vi "Popup - Select Operation.vi"(8 "error in (no error)":errorcluster, 11 "Controller (Host) Data in":T2={"State"=enum."APU Select", "2D User Info"=[], "APU Setup File"={"Sensor Info"=[], "Variables"=[], "CMM Table 106"=[], "CMM Table 106B "=[], "Accel Config"=[], "Report Sheet 1"=[], "Report Sheet 2"=[], "Report Sheet 3"=[]}, "Test Information"={"APU Part Number:"="", "Model:"="", "Serial Number:"="", "Customer:"="", "Work Order:"="", "Pre or Post SB"="", "Run Count"=0, "APU Selected"="<Select>"}, "ChannelTags"=[], "Live_Min_Max_Dev"=[], "CalChannels"=[], "Slopes"=[], "Offsets"=[], "Calculated Values"={"C.00"=0.0, "C.01"=0.0, "C.02"=0.0, "C.03"=0.0, "C.04"=0.0, "C.05"=0.0, "C.06"=0.0, "C.07"=0.0, "C.08"=0.0, "C.09"=0.0, "C.10"=0.0, "C.11"=0.0, "C.12"=0.0, "C.13"=0.0, "C.14"=0.0, "C.15"=0.0, "C.16"=0.0, "C.17"=0.0, "C.18"=0.0, "C.19"=0.0, "C.20"=0.0, "C.21"=0.0, "C.22"=0.0, "C.23"=0.0, "C.24"=0.0, "C.25"=0.0, "C.26"=0.0, "C.27"=0.0, "C.28"=0.0, "C.29"=0.0, "C.30"=0.0, "C.31"=0.0, "C.32"=0.0, "C.33"=0.0, "C.34"=0.0, "C.35"=0.0, "C.36"=0.0, "C.37"=0.0, "C.38"=0.0, "C.39"=0.0, "C.40"=0.0, "C.41"=0.0, "C.42"=0.0, "C.43"=0.0, "C.44"=0.0, "C.45"=0.0, "C.46"=0.0, "C.47"=0.0, "C.48"=0.0, "C.49"=0.0, "C.50"=0.0, "C.51"=0.0, "C.52"=0.0, "C.53"=0.0, "C.54"=0.0, "C.55"=0.0, "C.56"=0.0, "C.57"=0.0, "C.58"=0.0, "C.59"=0.0, "C.60"=0.0, "C.61"=0.0, "C.62"=0.0}, "ThresholdChannels"=[], "ThresholdRPM"=[], "ThresholdMin"=[], "ThresholdValue"=[], "HeavyCCM"=[], "LightCCM"=[], "FuelFarm"=FALSE} {"Test Information"."Run Count" min=0 step=1}) -> (0 "error out":errorcluster, 3 "Controller (Host) Data out":T2={"State"=enum."APU Select", "2D User Info"=[], "APU Setup File"={"Sensor Info"=[], "Variables"=[], "CMM Table 106"=[], "CMM Table 106B "=[], "Accel Config"=[], "Report Sheet 1"=[], "Report Sheet 2"=[], "Report Sheet 3"=[]}, "Test Information"={"APU Part Number:"="", "Model:"="", "Serial Number:"="", "Customer:"="", "Work Order:"="", "Pre or Post SB"="", "Run Count"=0, "APU Selected"="<Select>"}, "ChannelTags"=[], "Live_Min_Max_Dev"=[], "CalChannels"=[], "Slopes"=[], "Offsets"=[], "Calculated Values"={"C.00"=0.0, "C.01"=0.0, "C.02"=0.0, "C.03"=0.0, "C.04"=0.0, "C.05"=0.0, "C.06"=0.0, "C.07"=0.0, "C.08"=0.0, "C.09"=0.0, "C.10"=0.0, "C.11"=0.0, "C.12"=0.0, "C.13"=0.0, "C.14"=0.0, "C.15"=0.0, "C.16"=0.0, "C.17"=0.0, "C.18"=0.0, "C.19"=0.0, "C.20"=0.0, "C.21"=0.0, "C.22"=0.0, "C.23"=0.0, "C.24"=0.0, "C.25"=0.0, "C.26"=0.0, "C.27"=0.0, "C.28"=0.0, "C.29"=0.0, "C.30"=0.0, "C.31"=0.0, "C.32"=0.0, "C.33"=0.0, "C.34"=0.0, "C.35"=0.0, "C.36"=0.0, "C.37"=0.0, "C.38"=0.0, "C.39"=0.0, "C.40"=0.0, "C.41"=0.0, "C.42"=0.0, "C.43"=0.0, "C.44"=0.0, "C.45"=0.0, "C.46"=0.0, "C.47"=0.0, "C.48"=0.0, "C.49"=0.0, "C.50"=0.0, "C.51"=0.0, "C.52"=0.0, "C.53"=0.0, "C.54"=0.0, "C.55"=0.0, "C.56"=0.0, "C.57"=0.0, "C.58"=0.0, "C.59"=0.0, "C.60"=0.0, "C.61"=0.0, "C.62"=0.0}, "ThresholdChannels"=[], "ThresholdRPM"=[], "ThresholdMin"=[], "ThresholdValue"=[], "HeavyCCM"=[], "LightCCM"=[], "FuelFarm"=FALSE} {"Test Information"."Run Count" min=0 step=1})   [LabVIEW 2018, in "Controller (Host).lvlib"]
doc: "This is the dialog used by the user to select an operation to perform."
uses:
  Controller (Host).lvlib
  Private Controls/Controller (Host) Data.ctl
  Private Controls/State.ctl
  Top Level/Shared Controls/APU Setup File.ctl
  Public Controls/Test Information.ctl
  Public VIs/PreorPostSB.ctl
  Public Controls/APU Select.ctl
  Top Level/Shared Controls/Calculated Data.ctl
  File IO/Public Controls/Variables.ctl
  File IO/File IO.lvlib
  Testing UI 1/Testing UI 1.lvlib
panel:
  in  "Revert":bool
  in  "Variables":T1
  out "APU Selected":string
  in  "Confirm":bool
  # "Change APU Variables:"
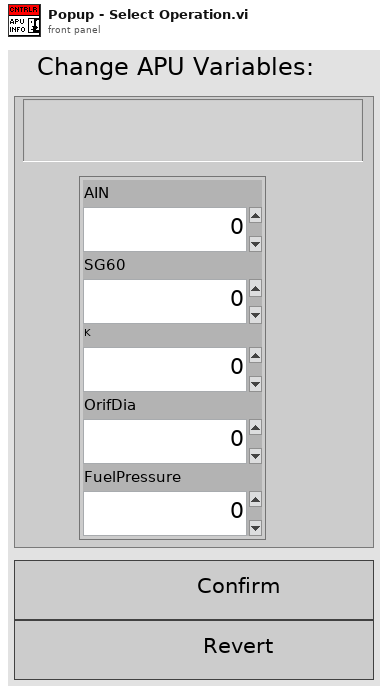
[diagram p1: front panel]
types:
  T1 = typedef "File IO.lvlib/Variables.ctl" = cluster{"AIN":dbl, "SG60":dbl, "K":dbl, "OrifDia":dbl, "FuelPressure":dbl}
  T2 = typedef "Controller (Host).lvlib/Controller (Host) Data.ctl" = cluster{"State":T3, "2D User Info":string[][], "APU Setup File":T4, "Test Information":T5, "ChannelTags":string[], "Live_Min_Max_Dev":dbl[][], "CalChannels":string[], "Slopes":dbl[], "Offsets":dbl[], "Calculated Values":T8, "ThresholdChannels":string[], "ThresholdRPM":dbl[], "ThresholdMin":bool[], "ThresholdValue":dbl[], "HeavyCCM":dbl[][], "LightCCM":dbl[][], "FuelFarm":bool}
  T3 = typedef "Controller (Host).lvlib/State.ctl" = enum16{"APU Select", "Operation Select", "SubTests Select", "Calibration", "Testing", "Exit"}
  T4 = typedef "APU Setup File.ctl" = cluster{"Sensor Info":string[][], "Variables":string[][], "CMM Table 106":string[][], "CMM Table 106B ":string[][], "Accel Config":string[][], "Report Sheet 1":string[][], "Report Sheet 2":string[][], "Report Sheet 3":string[][]}
  T5 = typedef "Controller (Host).lvlib/Test Information.ctl" = cluster{"APU Part Number:":string, "Model:":string, "Serial Number:":string, "Customer:":string, "Work Order:":string, "Pre or Post SB":T6, "Run Count":i32, "APU Selected":T7}
  T6 = typedef "Controller (Host).lvlib/PreorPostSB.ctl" = string
  T7 = typedef "Controller (Host).lvlib/APU Select.ctl" = string
  T8 = typedef "Calculated Data.ctl" = cluster{"C.00":dbl, "C.01":dbl, "C.02":dbl, "C.03":dbl, "C.04":dbl, "C.05":dbl, "C.06":dbl, "C.07":dbl, "C.08":dbl, "C.09":dbl, "C.10":dbl, "C.11":dbl, "C.12":dbl, "C.13":dbl, "C.14":dbl, "C.15":dbl, "C.16":dbl, "C.17":dbl, "C.18":dbl, "C.19":dbl, "C.20":dbl, "C.21":dbl, "C.22":dbl, "C.23":dbl, "C.24":dbl, "C.25":dbl, "C.26":dbl, "C.27":dbl, "C.28":dbl, "C.29":dbl, "C.30":dbl, "C.31":dbl, "C.32":dbl, "C.33":dbl, "C.34":dbl, "C.35":dbl, "C.36":dbl, "C.37":dbl, "C.38":dbl, "C.39":dbl, "C.40":dbl, "C.41":dbl, "C.42":dbl, "C.43":dbl, "C.44":dbl, "C.45":dbl, "C.46":dbl, "C.47":dbl, "C.48":dbl, "C.49":dbl, "C.50":dbl, "C.51":dbl, "C.52":dbl, "C.53":dbl, "C.54":dbl, "C.55":dbl, "C.56":dbl, "C.57":dbl, "C.58":dbl, "C.59":dbl, "C.60":dbl, "C.61":dbl, "C.62":dbl}
  T9 = cluster{"AIN":bool, "SG60":bool, "K":bool, "OrifDia":bool, "FuelPressure":bool}
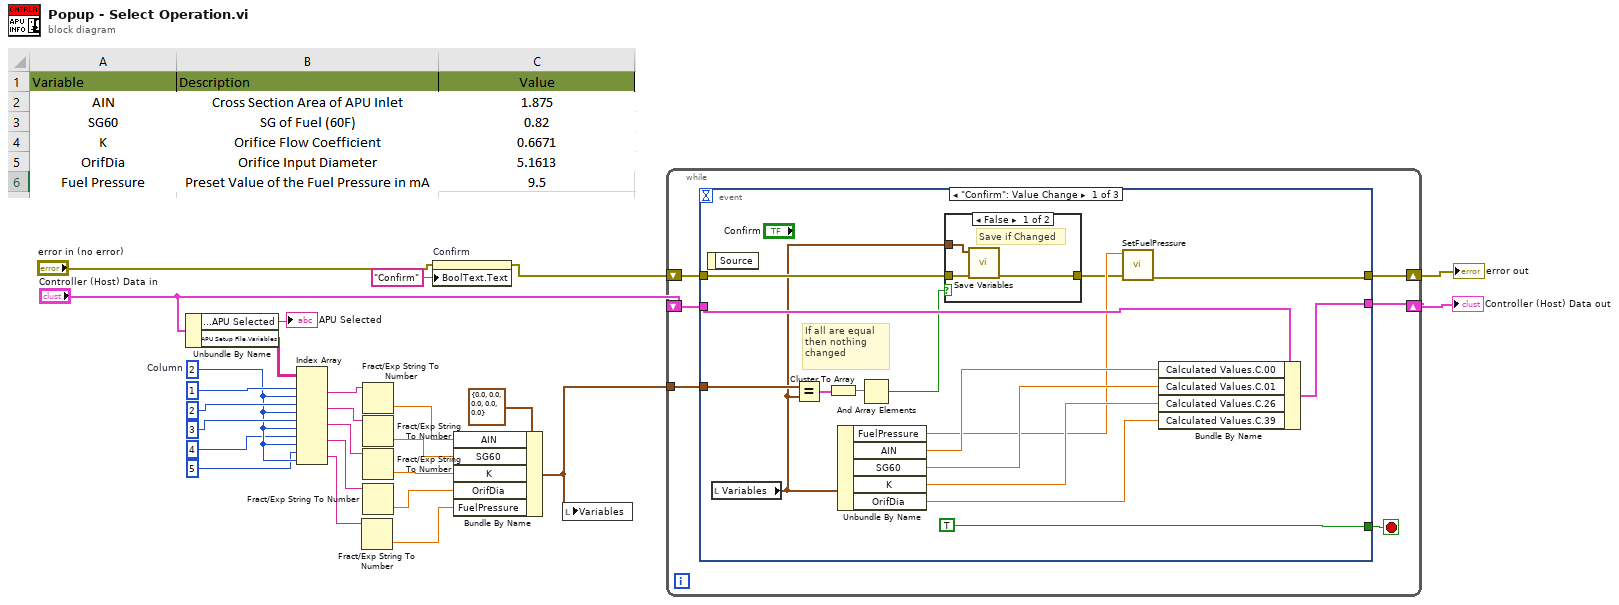
[diagram p0: block diagram]
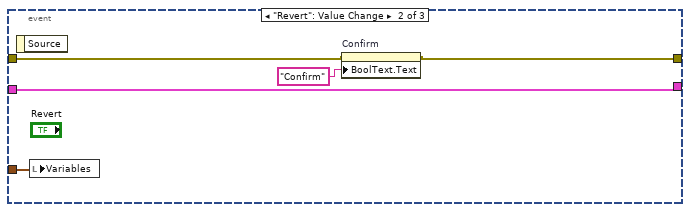
[diagram p3: hidden frame]
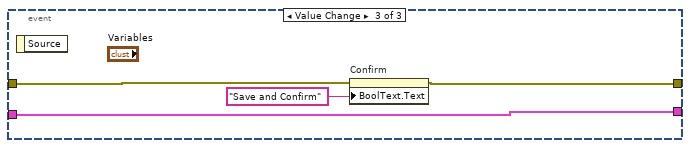
[diagram p4: hidden frame]
diagram:
  w18 = 2  # Column
  n1 = Unbundle By Name("Controller (Host) Data in") -> ("Test Information.APU Selected"=→"APU Selected":T7, "APU Setup File.Variables"=w23:string[][])
  n2 = Index Array(array=w23, index (row) #1=1 ("index (row)"), index (col) #1=w18, index (row) #2=2 ("index (row)"), index (col) #2=w18, index (row) #3=3 ("index (row)"), index (col) #3=w18, index (row) #4=4 ("index (row)"), index (col) #4=w18, index (row) #5=5 ("index (row)"), index (col) #5=w18) -> (element #1=w14:string, element #2=w12:string, element #3=w10:string, element #4=w9:string, element #5=w8:string)
  n3 = Fract/Exp String To Number(string=w8) -> (number=w5:dbl)  [unwired: 3 in, 1 out]
  n4 = Fract/Exp String To Number(string=w14) -> (number=w13:dbl)  [unwired: 3 in, 1 out]
  n5 = Fract/Exp String To Number(string=w12) -> (number=w11:dbl)  [unwired: 3 in, 1 out]
  n6 = Fract/Exp String To Number(string=w10) -> (number=w7:dbl)  [unwired: 3 in, 1 out]
  n7 = Fract/Exp String To Number(string=w9) -> (number=w6:dbl)  [unwired: 3 in, 1 out]
  n8 = property on="Confirm" class="Bool"(error in="error in (no error)", "BoolText.Text"="Confirm" ("Boolean Text.Text")) -> (error out=w2:errorcluster)  [unwired: 1 in, 1 out]
  n9 = Bundle By Name(cluster=T1 {"AIN"=0.0, "SG60"=0.0, "K"=0.0, "OrifDia"=0.0, "FuelPressure"=0.0} ("Variables"), "AIN"=w13, "SG60"=w11, "K"=w7, "OrifDia"=w6, "FuelPressure"=w5) -> (w4:T1)
  n10 = local write "Variables"(w4) -> ()
  n11 = while {
    shift-right: [w32] -> w25
    shift-left: "Controller (Host) Data in" -> [w31]
    shift-right: [w29] -> w24
    shift-left: w2 -> [w28]
    tunnel: w4 -> [w27]
    stop <- w30 stop-if-true
    n12 = event shown="[0] \"Confirm\": Value Change" {
      selector: _ -> [_ _ _]
      dyn-events: _ -> [_ _ _]
      timeout: _ -> [_ _ _]
      tunnel: [w46 w57 w61] -> w32
      tunnel: w31 -> [w47 w57 w61]
      tunnel: [TRUE _ _] -> w30
      tunnel: w28 -> [w38 w54 w60]
      tunnel: [w40 w53 w59] -> w29
      tunnel: w27 -> [w39 w56 _]
      event "Confirm": Value Change {
        # "If all are equal then nothing\nchanged"
        n13 = event-data() -> ()  [unwired: 1 in, 1 out]
        n14 = local read "Variables"() -> (w33:T1)
        n15 = Equal?(x=w39, y=w33) -> (x = y?=w36:T9)
        n16 = Cluster To Array(cluster=w36) -> (array=w35:bool[])
        n17 = Unbundle By Name(w33) -> ("FuelPressure"=w41:dbl, "AIN"=w45:dbl, "SG60"=w44:dbl, "K"=w43:dbl, "OrifDia"=w42:dbl)
        n18 = And Array Elements(Boolean array=w35) -> (logical AND=w34:bool)
        n19 = case shown="False" w34 {
          tunnel: w38 -> [w51 w52]
          tunnel: [w50 w52] -> w37
          tunnel: w33 -> [w49 _]
          frame False {
            # "Save if Changed"
            n20 = call "Save Variables.vi"("error in (no error)"=w51, "Variables"=w49) -> ("error out"=w50:errorcluster)  [unwired: 9 in]
          }
          frame True {
          }
        }
        n21 = call "SetFuelPressure.vi"("error in (no error)"=w37, "FuelPressure(ma)"=w41) -> ("error out"=w40:errorcluster)  [unwired: 9 in]
        n22 = Bundle By Name(cluster=w47, "Calculated Values.C.00"=w45, "Calculated Values.C.01"=w44, "Calculated Values.C.26"=w43, "Calculated Values.C.39"=w42) -> (w46:T2)
      }
      event "Revert": Value Change {
        n23 = event-data() -> ()  [unwired: 1 in, 1 out]
        n24 = local write "Variables"(w56) -> ()
        n25 = property on="Confirm" class="Bool"(error in=w54, "BoolText.Text"="Confirm" ("Boolean Text.Text")) -> (error out=w53:errorcluster)  [unwired: 1 in, 1 out]
      }
      event Value Change {
        n26 = event-data() -> ()  [unwired: 1 in, 1 out]
        n27 = property on="Confirm" class="Bool"(error in=w60, "BoolText.Text"="Save and Confirm" ("Boolean Text.Text")) -> (error out=w59:errorcluster)  [unwired: 1 in, 1 out]
      }
    }
  }
  "error out" <- w24
  "Controller (Host) Data out" <- w25
